vi "2-1 LabVIEW HTTP POST Request.vi"() -> ()   [LabVIEW 2020]
uses:
  <vilib>/httpClient/POSTBuffer.vi
  <vilib>/httpClient/LabVIEWHTTPClient.lvlib
panel:
  out "headers":string
  in  "error in":errorcluster
  out "error out":errorcluster
  out "body":string
  in  "flow":dbl=3.1
  in  "pressure":dbl=2.555
  in  "temperature":dbl=32.1
  in  "stop":bool
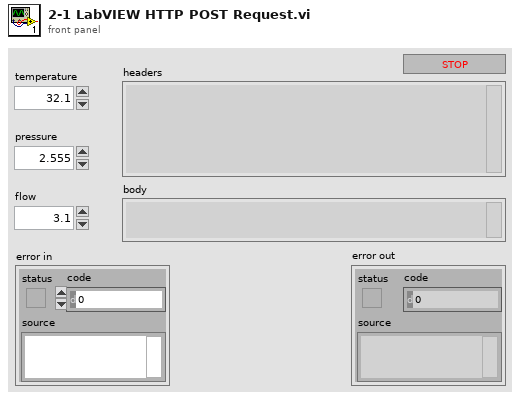
[diagram p1: front panel]
types:
  T1 = typedef "LabVIEWHTTPClient.lvlib/ClientHandle.ctl" = refnum<k1>
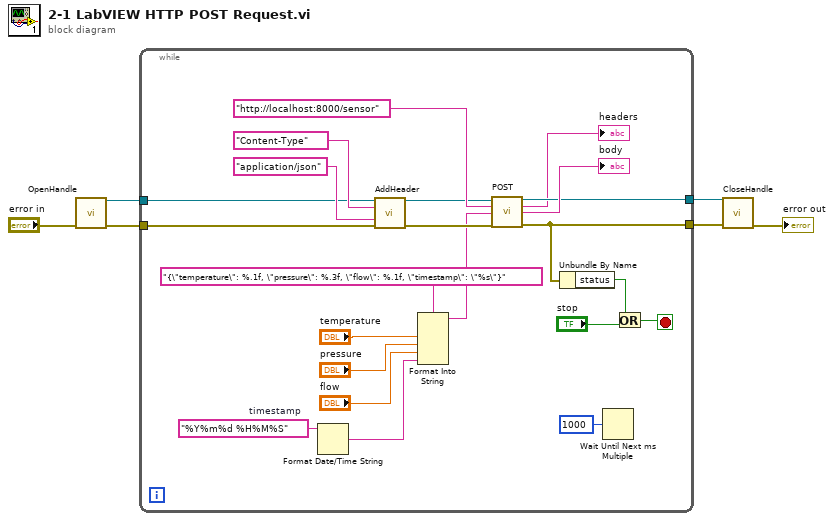
[diagram p0: block diagram]
diagram:
  n1 = call <vilib>:"OpenHandle.vi"("error in (no error)"="error in") -> ("client handle out"=w6:T1, "error out"=w5:errorcluster)  [unwired: 13 in]
  n2 = while {
    tunnel: w6 -> [w14]
    tunnel: w5 -> [w13]
    tunnel: [w12] -> w3
    tunnel: [w10] -> w2
    stop <- w7 stop-if-true
    w16 = "%Y%m%d %H%M%S"  # timestamp
    n3 = Format Date/Time String(time format string (%c)=w16) -> (date/time string=w17:string)  [unwired: 2 in]
    n4 = call <vilib>:"AddHeader.vi"("client handle"=w14, "header"="Content-Type", "value"="application/json", "error in (no error)"=w13) -> ("client handle out"=w27:T1, "error out"=w26:errorcluster)  [unwired: 10 in]
    n5 = Format Into String(format string="{\"temperature\": %.1f, \"pressure\": %.3f, \"flow\": %.1f, \"timestamp\": \"%s\"}", "temperature", "pressure", "flow", w17) -> (resulting string=w18:string)  [unwired: 2 in, 1 out]
    n6 = call-poly <vilib>:"POST.vi"("client handle"=w27, "url"="http://localhost:8000/sensor", "buffer"=w18, "error in (no error)"=w26) -> ("client handle out"=w12:T1, "headers"=→"headers":string, "body"=→"body":string, "error out"=w10:errorcluster)  [unwired: 8 in]
    n7 = Unbundle By Name(w10) -> ("status"=w9:bool)
    n8 = Wait Until Next ms Multiple(millisecond multiple=u32 1000) -> ()  [unwired: 1 out]
    n9 = Or(x=w9, y="stop") -> (x .or. y?=w7:bool)
  }
  n10 = call <vilib>:"CloseHandle.vi"("client handle"=w3, "error in (no error)"=w2) -> ("error out"=→"error out":errorcluster)  [unwired: 13 in]
